vi "Two sample t-test.vi"(4 "Significant level":enum16{"0.05", "0.01"}(ring), 5 "Alternate Hypothesis":enum16{"One-tailed", "Two-tailed"}(ring)=enum."Two-tailed", 6 "Data SET II":dbl[](array[numeric]), 7 "Data SET I":dbl[](array[numeric])) -> (2 "Reject null hypothesis":bool, 3 "t-Test Statistics":cluster{"t-Value":dbl, "DF":i32, "P-value":dbl})   [LabVIEW 2017]
uses:
  <vilib>/gmath/statdist.llb/Student t CDF.vi
  <vilib>/Analysis/NI_AALBase.lvlib
  <vilib>/gmath/NI_Gmath.lvlib
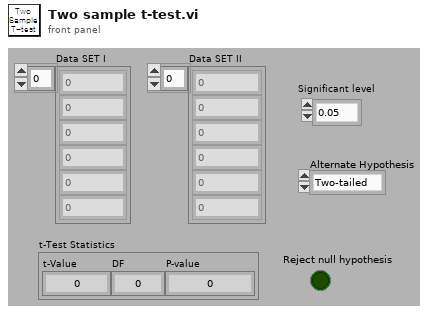
[diagram p1: front panel]
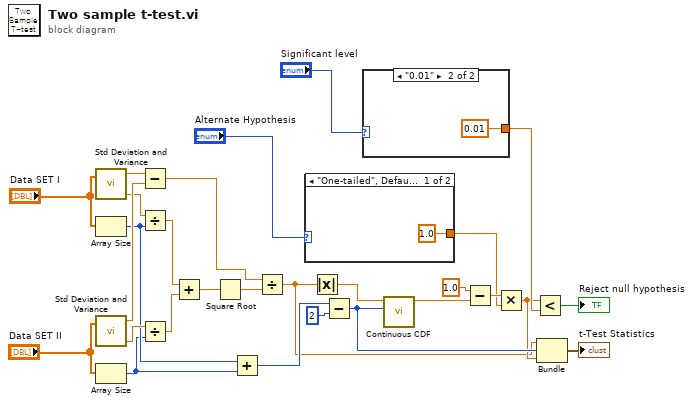
[diagram p0: block diagram]
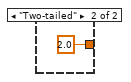
[diagram p2: hidden frame]
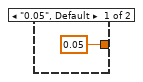
[diagram p3: hidden frame]
diagram:
  n1 = call <vilib>:"Std Deviation and Variance.vi"("X"="Data SET I") -> ("mean"=w26:dbl, "variance"=w23:dbl)  [unwired: 1 in, 1 out]
  n2 = Array Size(array="Data SET I") -> (size(s)=w17:i32)
  n3 = call <vilib>:"Std Deviation and Variance.vi"("X"="Data SET II") -> ("mean"=w25:dbl, "variance"=w22:dbl)  [unwired: 1 in, 1 out]
  n4 = Array Size(array="Data SET II") -> (size(s)=w16:i32)
  n5 = Subtract(x=w26, y=w25) -> (x-y=w24:dbl)
  n6 = Divide(x=w23, y=w17) -> (x/y=w20:dbl)
  n7 = Divide(x=w22, y=w16) -> (x/y=w21:dbl)
  n8 = Add(x=w20, y=w21) -> (x+y=w19:dbl)
  n9 = Square Root(x=w19) -> (sqrt(x)=w18:dbl)
  n10 = Add(x=w17, y=w16) -> (x+y=w15:i32)
  n11 = Divide(x=w24, y=w18) -> (x/y=w3:dbl)
  n12 = case shown="\"One-tailed\", Default" "Alternate Hypothesis" {
    tunnel: [1.0 ("x") 2.0 ("x")] -> w10
    frame "One-tailed", Default {
    }
    frame "Two-tailed" {
    }
  }
  n13 = Absolute Value(x=w3) -> (abs(x)=w2:dbl)
  n14 = Subtract(x=w15, y=2) -> (x-y=w6:i32)
  n15 = case shown="\"0.01\"" "Significant level" {
    tunnel: [0.05 0.01] -> w8
    frame "0.05", Default {
    }
    frame "0.01" {
    }
  }
  n16 = call-poly <vilib>:"Continuous CDF.vi"("k degrees of freedom"=w6, "x"=w2) -> ("cdf(x)"=w13:dbl)  [unwired: 7 in, 2 out]
  n17 = Subtract(x=1.0, y=w13) -> (x-y=w11:dbl)
  n18 = Multiply(x=w11, y=w10) -> (x*y=w5:dbl)
  n19 = Less?(x=w5, y=w8) -> (x < y?=→"Reject null hypothesis":bool)
  n20 = Bundle(w3, w6, w5) -> (→"t-Test Statistics":cluster{dbl, i32, dbl})  [unwired: 1 in]
